vi "e.gate HighSpeedPort Read Buffer State.vi"(8 "error in (no error)":errorcluster, 11 "Configuration in":T1) -> (0 "Error out":errorcluster caption="error out", 3 "Configuration out":T1)   [LabVIEW 2016]
doc: "This VI is used to receive and decode buffer state information's to the configuration cluster."
uses:
  e.gate Configuration.ctl
  e.gate Channel Data.ctl
  e.gate Data Type.ctl
  e.gate Protocol Type.ctl
  e.gate Module  Data.ctl
  e.gateHSP_DLLhandle.ctl
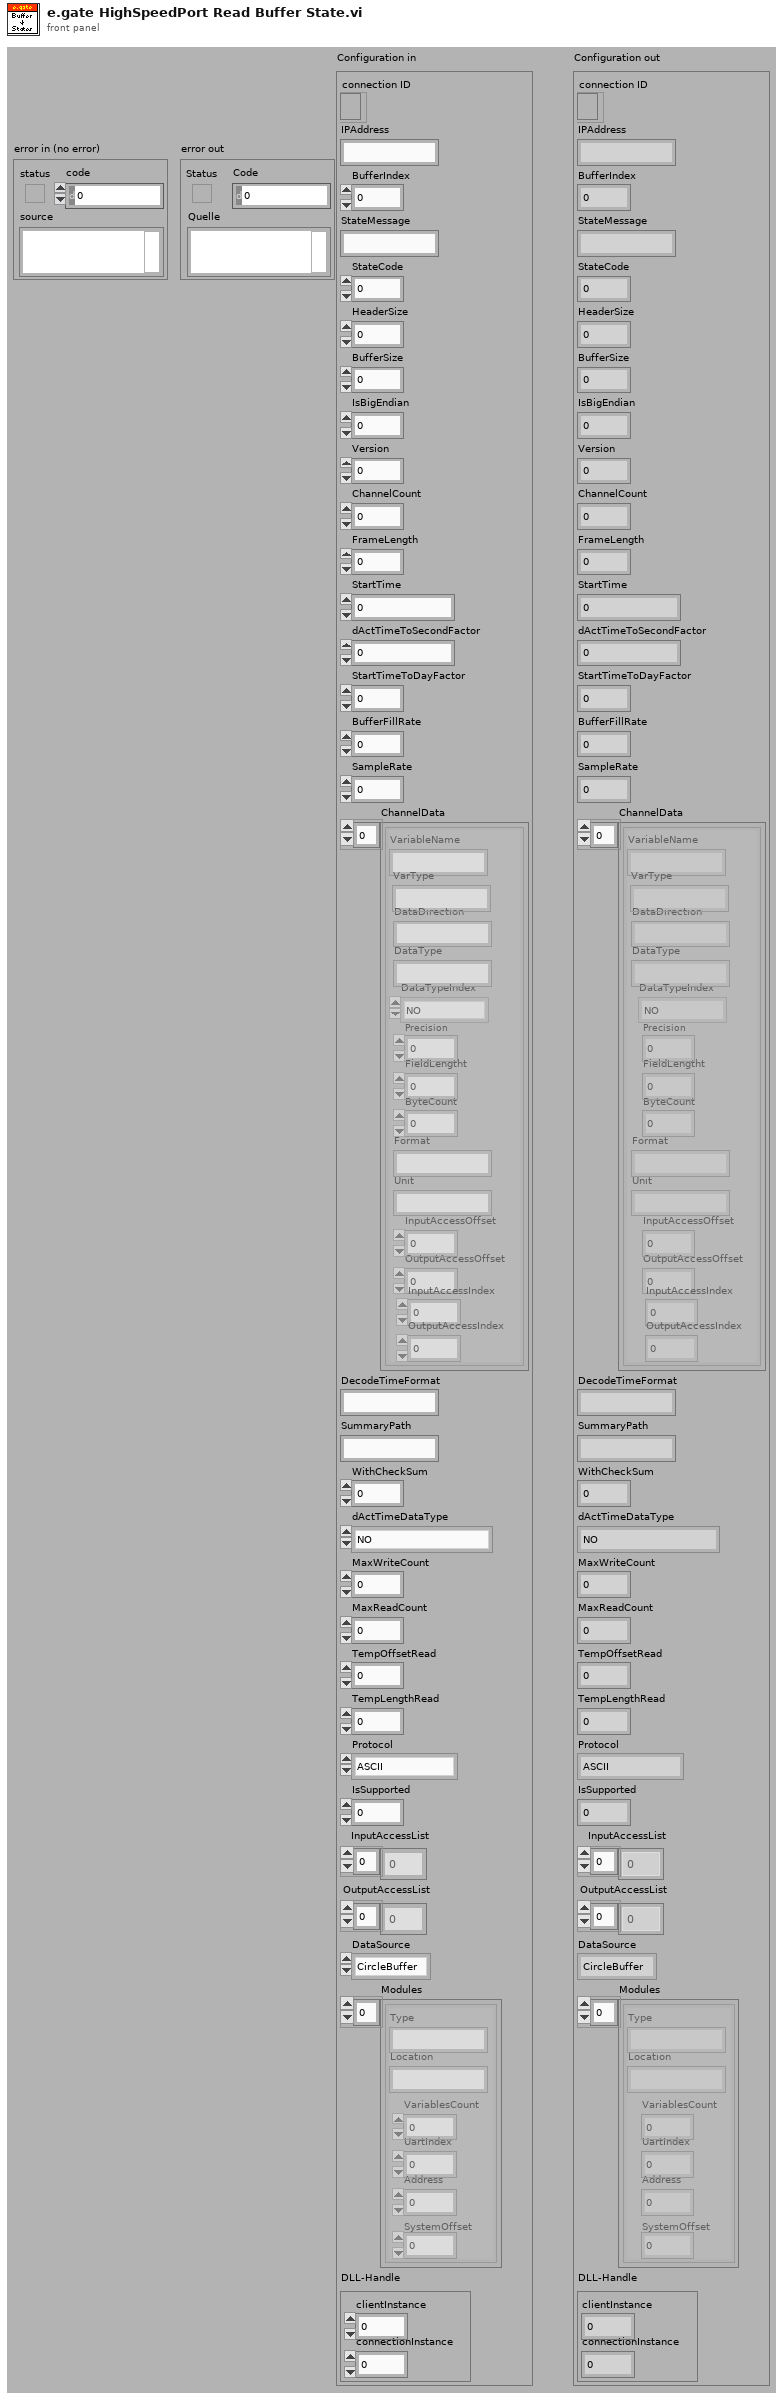
[diagram p1: front panel]
types:
  T1 = typedef "e.gate Configuration.ctl" = cluster{"connection ID":refnum<k5>, "IPAddress":string, "BufferIndex":i32, "StateMessage":string, "StateCode":i8, "HeaderSize":i32, "BufferSize":i32, "IsBigEndian":i32, "Version":i32, "ChannelCount":i32, "FrameLength":i32, "StartTime":dbl, "dActTimeToSecondFactor":dbl, "StartTimeToDayFactor":dbl, "BufferFillRate":dbl, "SampleRate":dbl, "ChannelData":T2[], "DecodeTimeFormat":string, "SummaryPath":string, "WithCheckSum":i32, "dActTimeDataType":T3, "MaxWriteCount":i32, "MaxReadCount":i32, "TempOffsetRead":i32, "TempLengthRead":i32, "Protocol":T4, "IsSupported":i32, "InputAccessList":i32[], "OutputAccessList":i32[], "DataSource":enum16{"CircleBuffer", "test.con Logger", "test.con Archive"}, "Modules":T5[], "DLL-Handle":T6}
  T2 = typedef "e.gate Channel Data.ctl" = cluster{"VariableName":string, "DataDirection":string, "DataType":string, "DataTypeIndex":T3, "Precision":i16, "FieldLengtht":i16, "ByteCount":i32, "Format":string, "Unit":string, "InputAccessOffset":i32, "OutputAccessOffset":i16, "InputAccessIndex":i16, "OutputAccessIndex":i16, "VarType":string}
  T3 = typedef "e.gate Data Type.ctl" = enum16{"NO", "BOOL", "SINT8", "USINT8", "SINT16", "USINT16", "SINT32", "USINT32", "FLOAT", "SET8", "SET16", "SET32", "DOUBLE", "SINT64", "USINT64", "SET64"}
  T4 = typedef "e.gate Protocol Type.ctl" = enum16{"ASCII", "HighspeedPort Online", "HighspeedPort Buffer", "eGateHighspeedPortDLL "}
  T5 = typedef "e.gate Module  Data.ctl" = cluster{"Type":string, "Location":string, "VariablesCount":i16, "UartIndex":i16, "Address":i16, "SystemOffset":i16}
  T6 = typedef "e.gateHSP_DLLhandle.ctl" = cluster{"clientInstance":i32, "connectionInstance":i32}
  T7 = enum16{"CircleBuffer", "test.con Logger", "test.con Archive"}
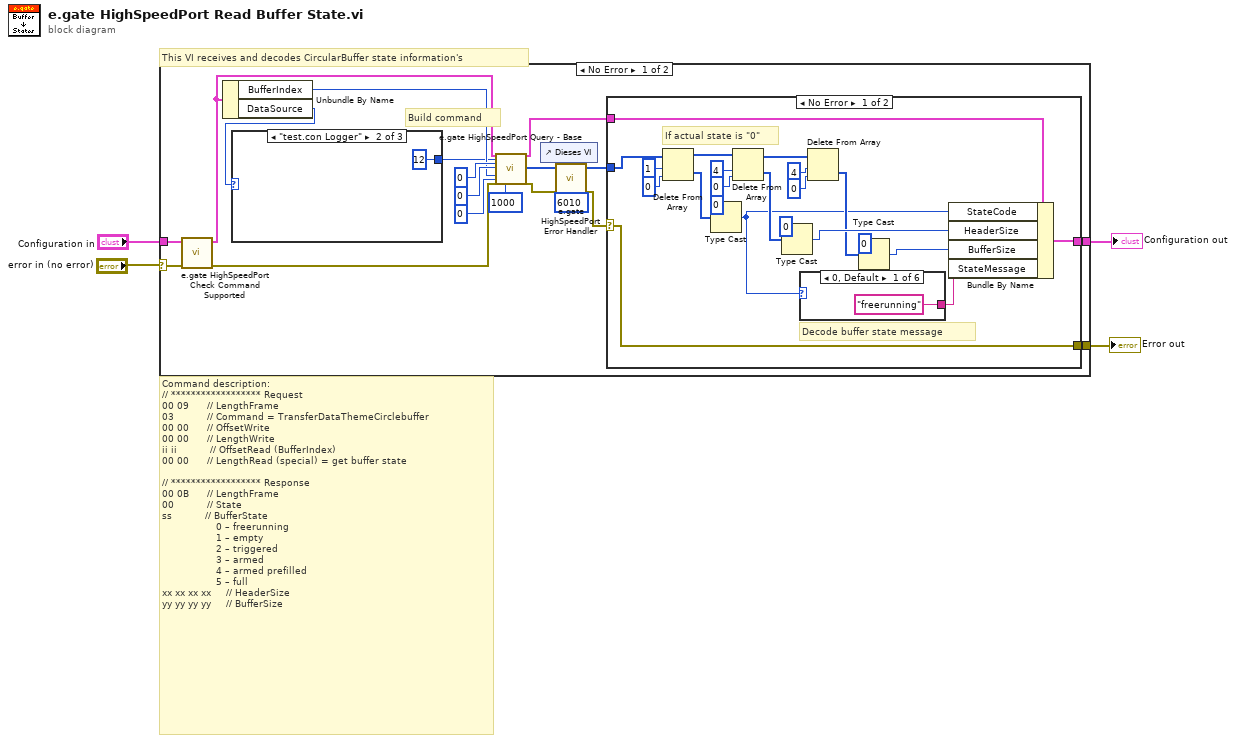
[diagram p0: block diagram]
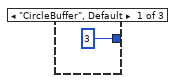
[diagram p2: hidden frame]
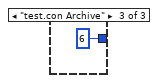
[diagram p3: hidden frame]
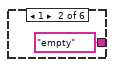
[diagram p4: hidden frame]
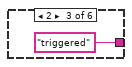
[diagram p5: hidden frame]
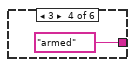
[diagram p6: hidden frame]
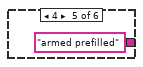
[diagram p7: hidden frame]
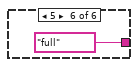
[diagram p8: hidden frame]
diagram:
  # "Command description:\n// ****************** Request\n00 09\t\t\t\t\t\t// LengthFrame\n03\t\t\t\t\t\t     // Command = TransferDataThemeCirclebuffer\n00 00\t\t\t\t\t\t// OffsetWrite\n00 00\t\t\t\t\t\t// LengthWrite\nii ii\t\t\t\t\t\t     // OffsetRead (BufferIndex)\n00 00\t\t\t\t\t\t// LengthRead (special) = get buffer state\n\n// ****************** Response\n00 0B\t\t\t\t\t\t// LengthFrame\n00\t\t\t\t\t\t    \t// State\nss\t\t\t\t\t\t     // BufferState\n\t\t\t\t\t\t\t          \t0 – freerunning\n\t\t\t\t\t\t          \t\t1 – empty\n\t\t\t\t\t\t\t          \t2 – triggered\n\t\t\t\t\t\t          \t\t3 – armed\n\t\t\t\t\t\t          \t\t4 – armed prefilled\n\t\t\t\t\t\t\t          \t5 – full\nxx xx xx xx\t\t\t\t\t// HeaderSize\nyy yy yy yy\t\t\t\t\t// BufferSize"
  # "This VI receives and decodes CircularBuffer state information's"
  n1 = case shown="No Error" "error in (no error)" {
    selector: "error in (no error)" -> [w18 w59]
    tunnel: [w7 w59] -> w3
    tunnel: [w19 w58] -> w4
    tunnel: "Configuration in" -> [w17 w58]
    frame No Error {
      # "Build command"
      n2 = call "e.gate HighSpeedPort Check Command Supported.vi"("error in (no error)"=w18, "Configuration in"=w17) -> ("error out"=w16:errorcluster, "Configuration out"=w15:T1)  [unwired: 8 out]
      n3 = Unbundle By Name(w15) -> ("BufferIndex"=w20:i32, "DataSource"=w6:T7)
      n4 = case shown="\"test.con Logger\"" w6 {
        tunnel: [3 ("Command") 12 ("Command") 6 ("Command")] -> w5
        frame "CircleBuffer", Default {
        }
        frame "test.con Logger" {
        }
        frame "test.con Archive" {
        }
      }
      n5 = call "e.gate HighSpeedPort Query - Base.vi"("e.gate Configuration in"=w15, "Command"=w5, "OffsetWrite"=0 ("Command"), "LengthWrite"=0 ("Command"), "OffsetRead"=w20, "LengthRead"=0 ("Command"), "error in (no error)"=w16, "Timeout (1000)"=1000) -> ("e.gate Configuration out"=w14:T1, "Data (out binary)"=w10:u8[], "error out"=w11:errorcluster)  [unwired: 2 in, 15 out]
      n6 = control-ref of="Dieses VI"() -> (w13:refnum<vi>)
      n7 = call "e.gate HighSpeedPort Error Handler.vi"("error code start index"=6010, "VI reference"=w13, "error in (no error)"=w11, "binary data in"=w10) -> ("error out"=w8:errorcluster, "binary out"=w9:u8[])  [unwired: 6 out]
      n8 = case shown="No Error" w8 {
        selector: w8 -> [w29 w57]
        tunnel: [w49 w56] -> w19
        tunnel: w14 -> [w48 w56]
        tunnel: w9 -> [w28 _]
        tunnel: [w29 w57] -> w7
        frame No Error {
          # "Decode buffer state message"
          # "If actual state is \"0\""
          n9 = Delete From Array(array=w28, length=1 ("Länge"), index=0 ("Index")) -> (deleted portion=w38:u8[], array with subset deleted=w44:u8[])
          n10 = Type Cast(type=i8 0, x=w38) -> (*(type *) &x=w31:i8)
          n11 = Delete From Array(array=w44, length=4 ("Länge"), index=0 ("Index")) -> (deleted portion=w36:u8[], array with subset deleted=w43:u8[])
          n12 = Type Cast(type=0, x=w36) -> (*(type *) &x=w35:i32)
          n13 = case shown="0, Default" w31 {
            tunnel: ["freerunning" "empty" "triggered" "armed" "armed prefilled" "full"] -> w30
            frame 0, Default {
            }
            frame 1 {
            }
            frame 2 {
            }
            frame 3 {
            }
            frame 4 {
            }
            frame 5 {
            }
          }
          n14 = Delete From Array(array=w43, length=4 ("Länge"), index=0 ("Index")) -> (deleted portion=w33:u8[])  [unwired: 1 out]
          n15 = Type Cast(type=0, x=w33) -> (*(type *) &x=w32:i32)
          n16 = Bundle By Name(cluster=w48, "StateCode"=w31, "HeaderSize"=w35, "BufferSize"=w32, "StateMessage"=w30) -> (w49:T1)
        }
        frame Error {
        }
      }
    }
    frame Error {
    }
  }
  "Error out" <- w3
  "Configuration out" <- w4
